vi "Rename Labels.vi"(8 "error in":errorcluster, 11 "Class Path":path) -> (0 "error out":errorcluster)   [LabVIEW 2020, in "PluginMetaDataObj.lvclass"]
doc: "This VI renames the Label of all the controls and indicators of VIs inside the class."
uses:
  PluginMetaDataObj.lvclass
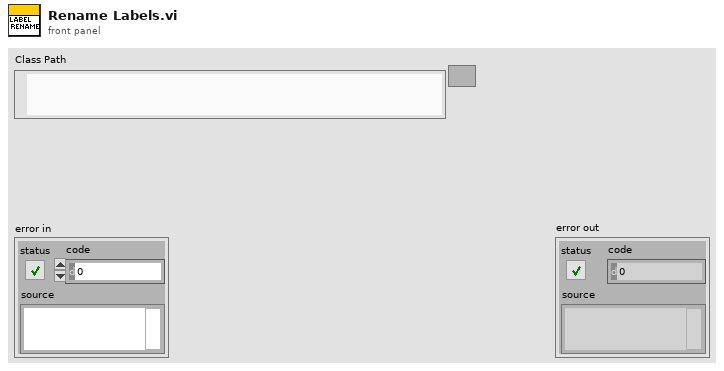
[diagram p1: front panel]
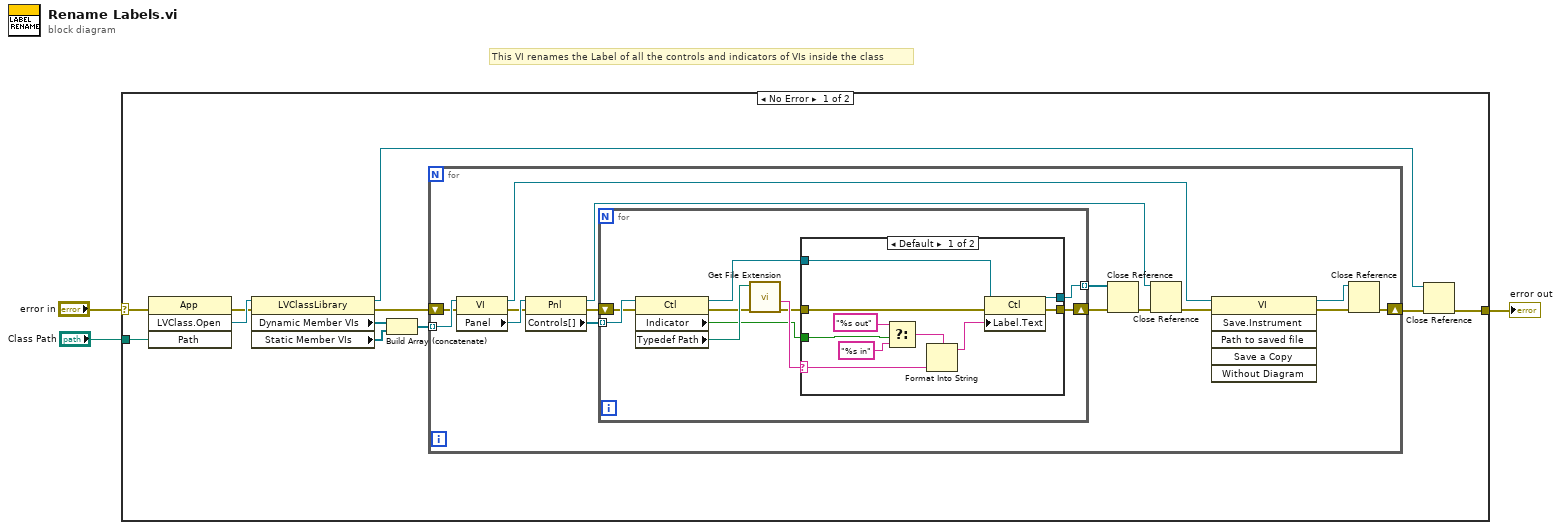
[diagram p0: block diagram]
diagram:
  # "This VI renames the Label of all the controls and indicators of VIs inside the class"
  n1 = case shown="No Error" "error in" {
    selector: "error in" -> [w13 w52]
    tunnel: [w14 w52] -> w3
    tunnel: "Class Path" -> [w4 _]
    frame No Error {
      n2 = invoke class="App" method="LVClass.Open"(error in=w13, "Path"=w4) -> (error out=w11:errorcluster, "LVClass.Open"=w12:refnum<vi>)  [unwired: 2 in, 2 out]
      n3 = property class="LVClassLibrary"(reference=w12, error in=w11) -> (reference out=w5:refnum<vi>, error out=w7:errorcluster, "Dynamic Member VIs"=w10:refnum<vi>[], "Static Member VIs"=w9:refnum<vi>[])
      n4 = Build Array (concatenate)(w10, w9) -> (w8:refnum<vi>[])
      n5 = for {
        tunnel: w8 -> [w17] mode=indexing
        shift-right: [w23] -> w6
        shift-left: w7 -> [w16]
        n6 = property class="VI"(reference=w17, error in=w16) -> (reference out=w20:refnum<vi>, error out=w18:errorcluster, "Panel"=w24:refnum<vi>)
        n7 = property class="Pnl"(reference=w24, error in=w18) -> (reference out=w29:refnum<vi>, error out=w25:errorcluster, "Controls[]"=w15:refnum<vi>[])
        n8 = for {
          tunnel: w15 -> [w36] mode=indexing
          shift-right: [w39] -> w26
          shift-left: w25 -> [w34]
          tunnel: [w38] -> w27 mode=indexing
          n9 = property class="Ctl"(reference=w36, error in=w34) -> (reference out=w35:refnum<vi>, error out=w31:errorcluster, "Indicator"=w32:bool, "Typedef Path"=w37:path)
          n10 = call <vilib>:"Get File Extension.vi"("error in (no error)"=w31, "file"=w37) -> ("error out"=w30:errorcluster, "filename without extension"=w33:string)  [unwired: 5 in, 3 out]
          n11 = case shown="Default" w33 {
            selector: w33 -> [w40 _]
            tunnel: w35 -> [w48 w50]
            tunnel: w30 -> [w44 w51]
            tunnel: [w43 w51] -> w39
            tunnel: [w42 w50] -> w38
            tunnel: w32 -> [w41 _]
            frame Default {
              n12 = Select(t="%s out", s=w41, f="%s in") -> (s? t:f=w45:string)
              n13 = Format Into String(format string=w45, w40) -> (resulting string=w49:string)  [unwired: 2 in, 1 out]
              n14 = property class="Ctl"(reference=w48, error in=w44, "Label.Text"=w49) -> (reference out=w42:refnum<vi>, error out=w43:errorcluster)
            }
            frame "" {
            }
          }
        }
        n15 = Close Reference(reference=w27, error in (no error)=w26) -> (error out=w28:errorcluster)
        n16 = Close Reference(reference=w29, error in (no error)=w28) -> (error out=w22:errorcluster)
        n17 = invoke class="VI" method="Save.Instrument"(reference=w20, error in=w22) -> (reference out=w19:refnum<vi>, error out=w21:errorcluster)  [unwired: 4 in, 4 out]
        n18 = Close Reference(reference=w19, error in (no error)=w21) -> (error out=w23:errorcluster)
      }
      n19 = Close Reference(reference=w5, error in (no error)=w6) -> (error out=w14:errorcluster)
    }
    frame Error {
    }
  }
  "error out" <- w3
